vi "downsample 1D array - U64.vi"(2 "Ave N":dbl, 3 "Array In":u64[](array[numeric])) -> (1 "Array Out":u64[](array[numeric]))   [LabVIEW 2014]
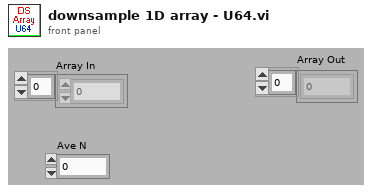
[diagram p1: front panel]
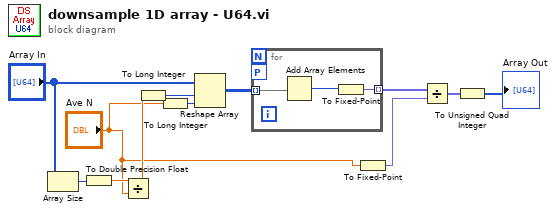
[diagram p0: block diagram]
diagram:
  n1 = Array Size(array="Array In") -> (size(s)=w12:i32)
  n2 = To Double Precision Float(number=w12) -> (double precision float=w8:dbl)
  n3 = Divide(x=w8, y="Ave N") -> (x/y=w11:dbl)
  n4 = To Long Integer(number=w11) -> (32bit integer=w7:i32)
  n5 = To Long Integer(number="Ave N") -> (32bit integer=w6:i32)
  n6 = Reshape Array("Array In", w7, w6) -> (w10:u64[][])
  n7 = for {
    tunnel: w10 -> [w15] mode=indexing
    workers-P: _ -> [_]
    tunnel: [w13] -> w4 mode=indexing
    n8 = Add Array Elements(numeric array=w15) -> (sum=w14:u64)
    n9 = To Fixed-Point(number=w14) -> (fixed-point=w13:fxp<+,64,64>)  [unwired: 1 in]
  }
  n10 = To Fixed-Point(number="Ave N") -> (fixed-point=w2:fxp<+,64,64>)  [unwired: 1 in]
  n11 = Divide(x=w4, y=w2) -> (x/y=w1:fxp<+,64,64>[])
  n12 = To Unsigned Quad Integer(1:w1) -> (0:→"Array Out":u64[])
